vi "Drawing a Circle.vi"(10 "number of points":i32=180, 11 "circle":cluster{"x0":dbl, "y0":dbl, "r":dbl}) -> (3 "circle graph":cluster{"x":dbl[], "y":dbl[]})   [LabVIEW 2023]
doc: "Convert a circle x0, y0, and r values into arrays of X and Y values that can be used to draw a circle in an XY Graph."
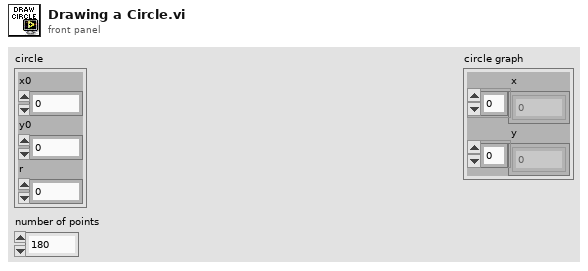
[diagram p1: front panel]
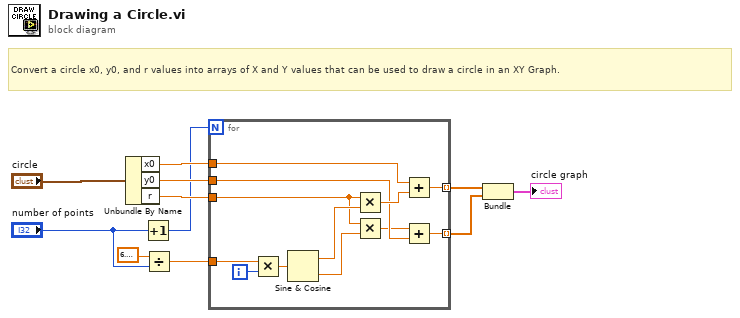
[diagram p0: block diagram]
diagram:
  # "Convert a circle x0, y0, and r values into arrays of X and Y values that can be used to draw a circle in an XY Graph."
  n1 = Unbundle By Name("circle") -> ("x0"=w5:dbl, "y0"=w3:dbl, "r"=w4:dbl)
  n2 = Increment(x="number of points") -> (x+1=w2:i32)
  n3 = Divide(x=6.283185307179586, y="number of points") -> (x/y=w9:dbl)
  n4 = for {
    N: w2 -> [_]
    tunnel: w9 -> [w23]
    tunnel: w4 -> [w18]
    tunnel: w5 -> [w17]
    tunnel: w3 -> [w15]
    tunnel: [w13] -> w8 mode=indexing
    tunnel: [w12] -> w7 mode=indexing
    i -> [w22]
    n5 = Multiply(x=w23, y=w22) -> (x*y=w21:dbl)
    n6 = Sine & Cosine(0:w21) -> (1:w20:dbl, 2:w19:dbl)
    n7 = Multiply(x=w18, y=w20) -> (x*y=w16:dbl)
    n8 = Multiply(x=w18, y=w19) -> (x*y=w14:dbl)
    n9 = Add(x=w17, y=w16) -> (x+y=w13:dbl)
    n10 = Add(x=w14, y=w15) -> (x+y=w12:dbl)
  }
  n11 = Bundle(w8, w7) -> (→"circle graph":cluster{dbl[], dbl[]})  [unwired: 1 in]
